vi "Read.vi"(2 "error in (no error)":errorcluster) -> (0 "error out":errorcluster, 1 "Numeric Out":i16)   [LabVIEW 2017]
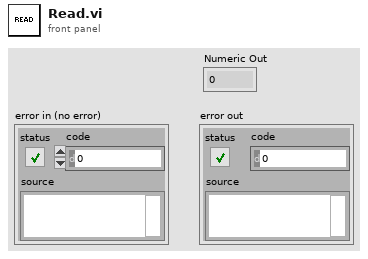
[diagram p1: front panel]
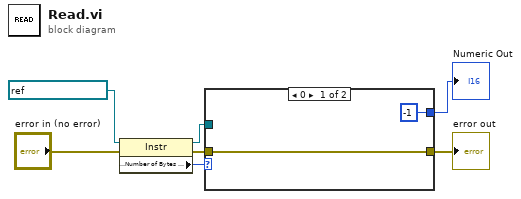
[diagram p0: block diagram]
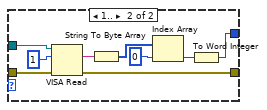
[diagram p2: hidden frame]
diagram:
  n1 = property class="Instr"(reference=refnum<visa-resource-name> "ASRL1::INSTR", error in="error in (no error)") -> (reference out=w2:refnum<visa-resource-name>, error out=w3:errorcluster, "Serial Settings:Number of Bytes at Serial Port"=w7:u32)
  n2 = case shown="0" w7 {
    tunnel: w2 -> [_ w18]
    tunnel: w3 -> [w9 w17]
    tunnel: [w9 w16] -> w4
    tunnel: [i16 -1 w10] -> w1
    frame 0 {
    }
    frame 1.. {
      n3 = VISA Read(VISA resource name=w18, byte count=u32 1, error in (no error)=w17) -> (read buffer=w15:string, error out=w16:errorcluster)  [unwired: 2 out]
      n4 = String To Byte Array(string=w15) -> (unsigned byte array=w14:u8[])
      n5 = Index Array(array=w14, index=0) -> (element=w11:u8)
      n6 = To Word Integer(number=w11) -> (16bit integer=w10:i16)
    }
  }
  "error out" <- w4
  "Numeric Out" <- w1
